vi "Create.vi"(8 "error in (no error)":errorcluster, 10 "Owner":refnum<vi>, 11 "Actor in":refnum<class "Actor.lvclass">) -> (0 "error out":errorcluster, 3 "API out":refnum<class "Interface.lvclass">)   [LabVIEW 2018, in "Scripting.lvlib" / "Actor.lvlib" / "Interface.lvclass"]
uses:
  Interface.lvclass
  Actor.lvclass
  Request-Enqueuers.ctl
  Get State.ctl
  State.ctl
  Stop.ctl
  Front-Panel State.ctl
  Actor-Stopped.ctl
  Interface.lvclass/Interface.ctl
  Actor-Caller.vi
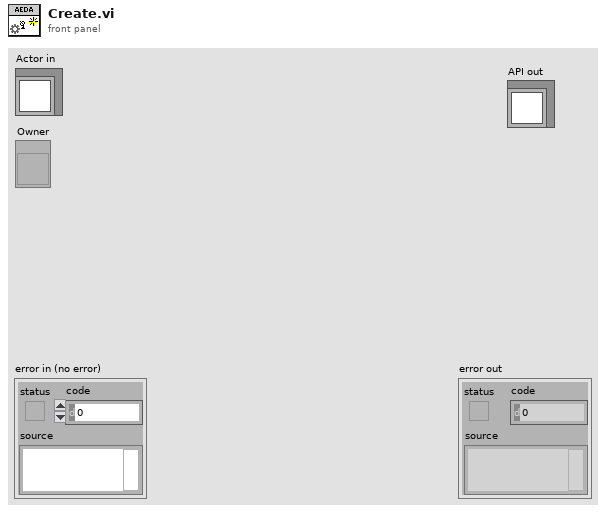
[diagram p1: front panel]
types:
  T1 = typedef "Scripting.lvlib/Actor.lvlib/Actor.lvclass/Front-Panel State.ctl" = enum16{"Don't Show", "Show"}
  T2 = typedef "Scripting.lvlib/Actor.lvlib/Actor.lvclass/Request-Enqueuers.ctl" = cluster{"Get State":refnum<user-event>, "Stop":refnum<user-event>}
  T3 = typedef "Scripting.lvlib/Actor.lvlib/Interface.lvclass/Actor-Stopped.ctl" = cluster{"Final State":refnum<class "Actor.lvclass">, "Final Error":errorcluster}
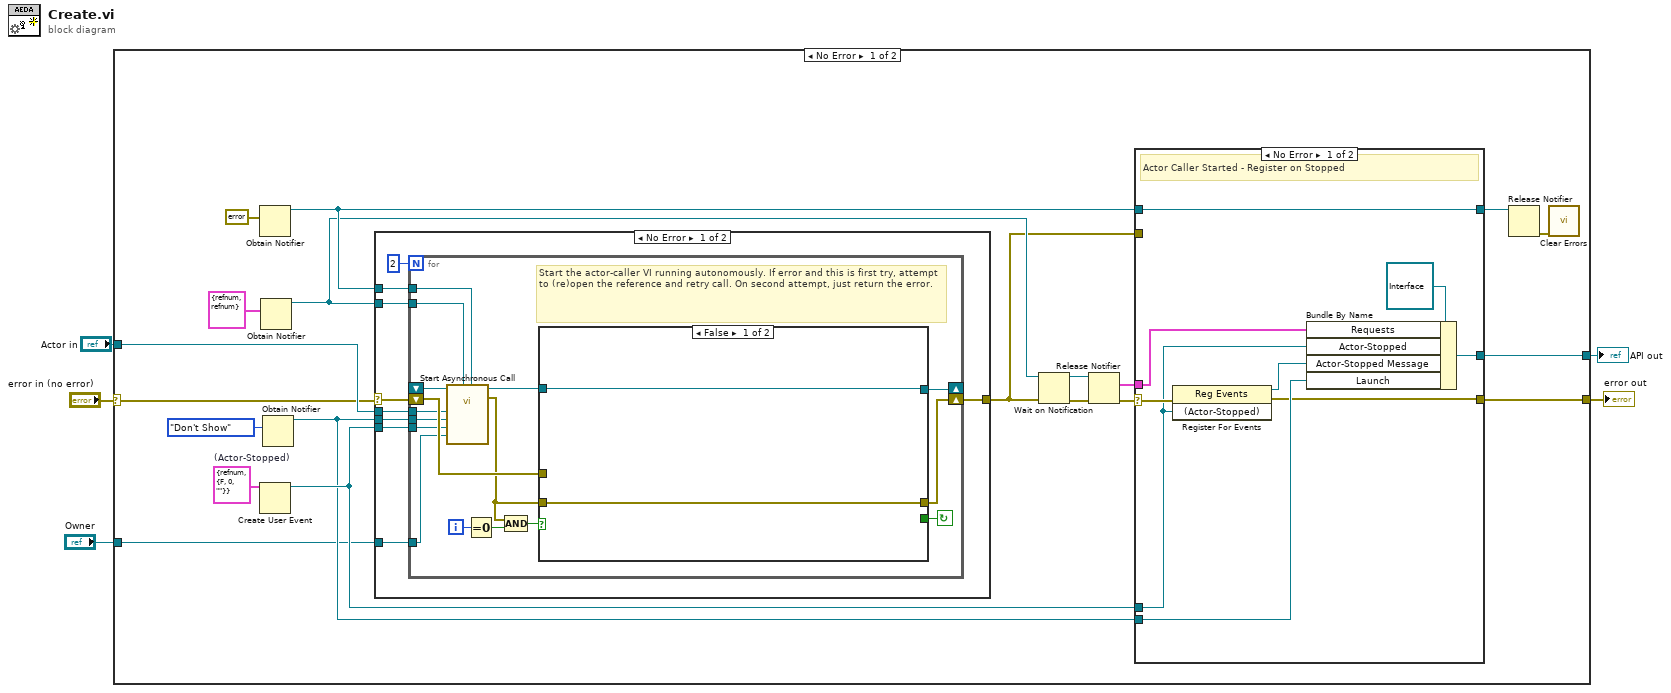
[diagram p0: block diagram]
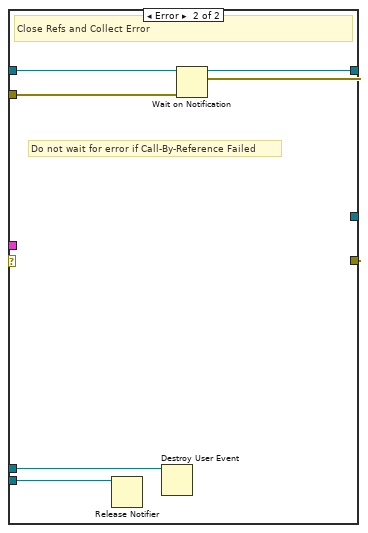
[diagram p2: hidden frame]
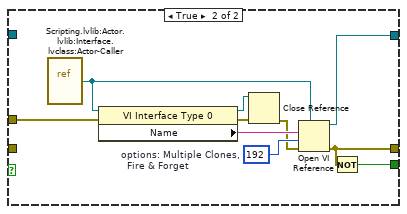
[diagram p3: hidden frame]
diagram:
  n1 = case shown="No Error" "error in (no error)" {
    selector: "error in (no error)" -> [w18 w79]
    tunnel: [w23 w79] -> w4
    tunnel: "Actor in" -> [w21 _]
    tunnel: [w16 _] -> w1
    tunnel: "Owner" -> [w12 _]
    frame No Error {
      w6 = T3 {"Final State"=refnum, "Final Error"={"status"=FALSE, "code"=0, "source"=""}}  # (Actor-Stopped)
      n2 = Obtain Notifier(notification data type=errorcluster {"status"=FALSE, "code"=0, "source"=""} ("error constant")) -> (notifier out=w22:refnum<notifier>)  [unwired: 3 in, 2 out]
      n3 = Create User Event(user event datatype=w6) -> (user event=w17:refnum<user-event>)  [unwired: 1 in, 1 out]
      n4 = Obtain Notifier(notification data type=T2 {"Get State"=refnum, "Stop"=refnum} ("Actor-Events")) -> (notifier out=w19:refnum<notifier>)  [unwired: 3 in, 2 out]
      n5 = Obtain Notifier(notification data type=Front-Panel_State."Don't Show" ("Front Panel State")) -> (notifier out=w15:refnum<notifier>)  [unwired: 3 in, 2 out]
      n6 = case shown="No Error" w18 {
        selector: w18 -> [w47 w78]
        tunnel: [w48 w78] -> w7
        tunnel: w19 -> [w46 _]
        tunnel: w22 -> [w45 _]
        tunnel: w21 -> [w44 _]
        tunnel: w15 -> [w43 _]
        tunnel: w17 -> [w42 _]
        tunnel: w12 -> [w41 _]
        frame No Error {
          n7 = for {
            N: 2 -> [_]
            shift-right: [w65] -> w48
            shift-left: w47 -> [w60]
            shift-right: [w59] -> _
            shift-left: _ -> [w58]
            tunnel: w46 -> [w52]
            tunnel: w45 -> [w51]
            tunnel: w44 -> [w55]
            tunnel: w43 -> [w54]
            tunnel: w42 -> [w53]
            tunnel: w41 -> [w50]
            i -> [w62]
            stop <- w61 continue-if-true
            # "Start the actor-caller VI running autonomously. If error and this is first try, attempt to (re)open the reference and retry call. On second attempt, just return the error."
            n8 = call-by-ref "Start Asynchronous Call"(reference=w58, "Initialize-Error Passback"=w51, "Enqueuers Passback"=w52, "Owner"=w50, "Stopped Enqueuer"=w53, "Launch"=w54, "Actor in"=w55) -> (reference out=w57:refnum<vi>, error out=w56:errorcluster)  [unwired: 7 in]
            n9 = Equal To 0?(x=w62) -> (x = 0?=w63:bool)
            n10 = Compound Arithmetic op=AND(w56, w63) -> (w64:bool)
            n11 = case shown="False" w64 {
              tunnel: [w66 w74] -> w59
              tunnel: [w67 w76] -> w65
              tunnel: w56 -> [w67 _]
              tunnel: [_ w77] -> w61
              tunnel: w60 -> [_ w75]
              tunnel: w57 -> [w66 _]
              frame False {
              }
              frame True {
                w72 = 192  # options: Multiple Clones,   Fire & Forget
                n12 = vi-ref "Scripting.lvlib:Actor.lvlib:Interface.lvclass:Actor-Caller.vi"() -> (w68:refnum<vi>)
                n13 = property class="VI Interface Type 0"(reference=w68, error in=w75) -> (reference out=w70:refnum<vi>, error out=w71:errorcluster, "Name"=w73:string)
                n14 = Close Reference(reference=w70, error in (no error)=w71) -> (error out=w69:errorcluster)
                n15 = Open VI Reference(type specifier VI Refnum (for type only)=w68, vi path=w73, options=w72, error in (no error)=w69) -> (vi reference=w74:refnum<vi>, error out=w76:errorcluster)  [unwired: 2 in]
                n16 = Not(x=w76) -> (.not. x?=w77:bool)
              }
            }
          }
        }
        frame Error {
        }
      }
      n17 = Wait on Notification(notifier=w19, error in (no error)=w7) -> (notifier out=w11:refnum<notifier>, error out=w10:errorcluster)  [unwired: 2 in, 2 out]
      n18 = Release Notifier(notifier=w11, error in (no error)=w10) -> (last notification=w8:T2, error out=w9:errorcluster)  [unwired: 1 in, 1 out]
      n19 = case shown="No Error" w9 {
        selector: w9 -> [w33 _]
        tunnel: w8 -> [w31 _]
        tunnel: w22 -> [w34 w40]
        tunnel: [w34 w39] -> w24
        tunnel: [w28 w38] -> w23
        tunnel: w17 -> [w30 w37]
        tunnel: w15 -> [w32 w36]
        tunnel: [w27 _] -> w16
        tunnel: w7 -> [_ w35]
        frame No Error {
          # "Actor Caller Started - Register on Stopped"
          n20 = register-events(error in=w33, w30) -> (reference out=w26:refnum<event-registration>, error out=w28:errorcluster)  [unwired: 1 in]
          n21 = Bundle By Name(cluster=refnum<class "Interface.lvclass"> refnum ("Scripting.lvlib:Actor.lvlib:Interface.lvclass"), "Requests"=w31, "Actor-Stopped"=w30, "Actor-Stopped Message"=w26, "Launch"=w32) -> (w27:refnum<class "Interface.lvclass">)
        }
        frame Error {
          # "Do not wait for error if Call-By-Reference Failed"
          # "Close Refs and Collect Error"
          n22 = Release Notifier(notifier=w36) -> ()  [unwired: 2 in, 3 out]
          n23 = Destroy User Event(user event=w37) -> ()  [unwired: 1 in, 1 out]
          n24 = Wait on Notification(notifier=w40, error in (no error)=w35) -> (notifier out=w39:refnum<notifier>, notification=w38:errorcluster)  [unwired: 2 in, 2 out]
        }
      }
      n25 = Release Notifier(notifier=w24) -> (error out=w13:errorcluster)  [unwired: 2 in, 2 out]
      n26 = call <vilib>:"Clear Errors.vi"("error in (no error)"=w13) -> ()  [unwired: 5 in, 2 out]
    }
    frame Error {
    }
  }
  "error out" <- w4
  "API out" <- w1
